vi "Do_Parameters_tl.vi"(2 "CHANNEL PARAMETERS":string[][](table), 5 "Axis Name":string) -> (1 "Current Axis Name":string)   [LabVIEW 2010]
panel:
  out "Axis Row":string[](array[string])
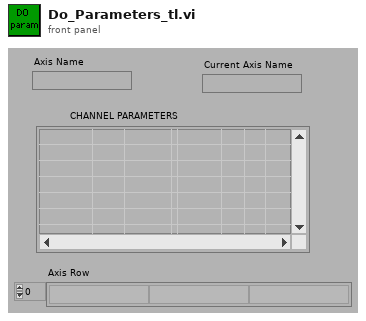
[diagram p1: front panel]
types:
  T1 = enum16{"Is Axis Current axis?", "Write Parameters", "Set Address", "Selected OK?", "Update current axis"}
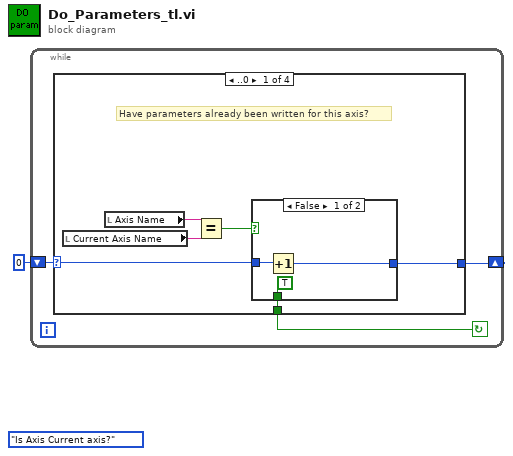
[diagram p0: block diagram]
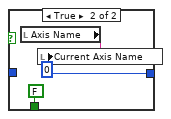
[diagram p2: hidden frame]
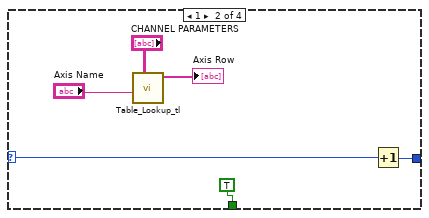
[diagram p3: hidden frame]
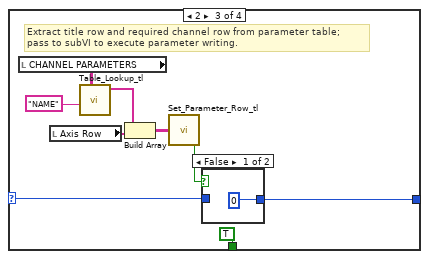
[diagram p4: hidden frame]
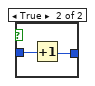
[diagram p5: hidden frame]
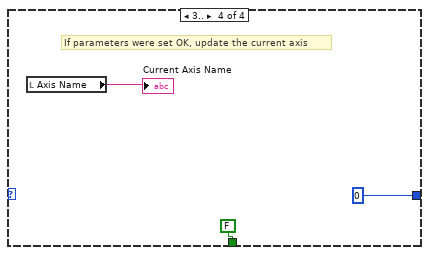
[diagram p6: hidden frame]
diagram:
  (unwired) T1."Is Axis Current axis?"
  n1 = while {
    shift-left: 0 -> [w4]
    shift-right: [w3] -> _
    stop <- w2 continue-if-true
    n2 = case shown="..0" w4 {
      selector: w4 -> [w8 w22 w26 _]
      tunnel: [w7 w21 w25 0] -> w3
      tunnel: [w6 TRUE TRUE FALSE] -> w2
      frame ..0 {
        # "Have parameters already been written for this axis?"
        n3 = local read "Current Axis Name"() -> (w9:string)
        n4 = local read "Axis Name"() -> (w10:string)
        n5 = Equal?(x=w10, y=w9) -> (x = y?=w5:bool)
        n6 = case shown="False" w5 {
          tunnel: w8 -> [w13 _]
          tunnel: [w12 0] -> w7
          tunnel: [TRUE FALSE] -> w6
          frame False {
            n7 = Increment(x=w13) -> (x+1=w12:i32)
          }
          frame True {
            n8 = local read "Axis Name"() -> (w14:string)
            n9 = local write "Current Axis Name"(w14) -> ()
          }
        }
      }
      frame 1 {
        n10 = call "Table_Lookup_tl.vi"("Lookup Table"="CHANNEL PARAMETERS", "Search String"="Axis Name") -> ("Output row"=→"Axis Row":string[])  [unwired: 3 in, 3 out]
        n11 = Increment(x=w22) -> (x+1=w21:i32)
      }
      frame 2 {
        # "Extract title row and required channel row from parameter table;\npass to subVI to execute parameter writing."
        n12 = local read "CHANNEL PARAMETERS"() -> (w31:string[][])
        n13 = local read "Axis Row"() -> (w29:string[])
        n14 = call "Table_Lookup_tl.vi"("Lookup Table"=w31, "Search String"="NAME") -> ("Output row"=w23:string[])  [unwired: 3 in, 3 out]
        n15 = Build Array(w23, w29) -> (w28:string[][])
        n16 = call "Set_Parameter_Row_tl.vi"("Parameter Row"=w28) -> ("PARAMETERS\nWRITTEN OK?"=w27:bool)  [unwired: 4 in]
        n17 = case shown="False" w27 {
          tunnel: w26 -> [_ w34]
          tunnel: [0 w33] -> w25
          frame False {
          }
          frame True {
            n18 = Increment(x=w34) -> (x+1=w33:i32)
          }
        }
      }
      frame 3.. {
        # "If parameters were set OK, update the current axis"
        n19 = local read "Axis Name"() -> (→"Current Axis Name":string)
      }
    }
  }
